vi "IMAQ_symmetrytransform_evenodd.vi"(4 "Destructive":bool, 5 "Optional Rectangle":i32[](array[numeric]), 6 "error in (no error)":errorcluster, 7 "margin":i32=15, 9 "Image Src":T1) -> (0 "error out":errorcluster, 2 "Centroid":cluster{"X Centroid":sgl, "Y Centroid":sgl} {"Y Centroid" format="%.2f"; "X Centroid" format="%.2f"}, 3 "Image Src Dup":T1)   [LabVIEW 2010]
uses:
  <vilib>/vision/Image Controls.llb/IMAQ Image.ctl
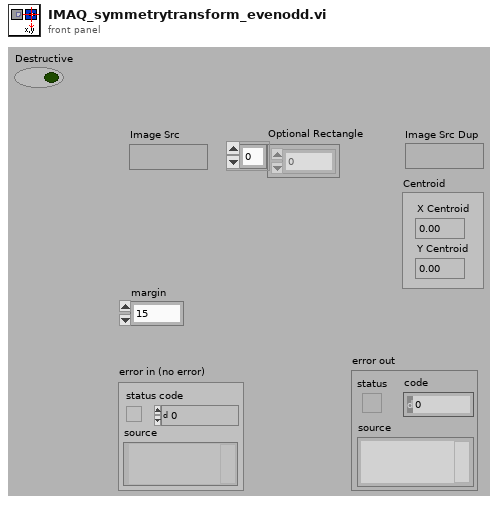
[diagram p1: front panel]
types:
  T1 = typedef "IMAQ Image.ctl" = refnum<image>
  T2 = enum32{"Map Pixel Pointer", "Unmap Pixel Pointer", "Get Pixels Infos"}
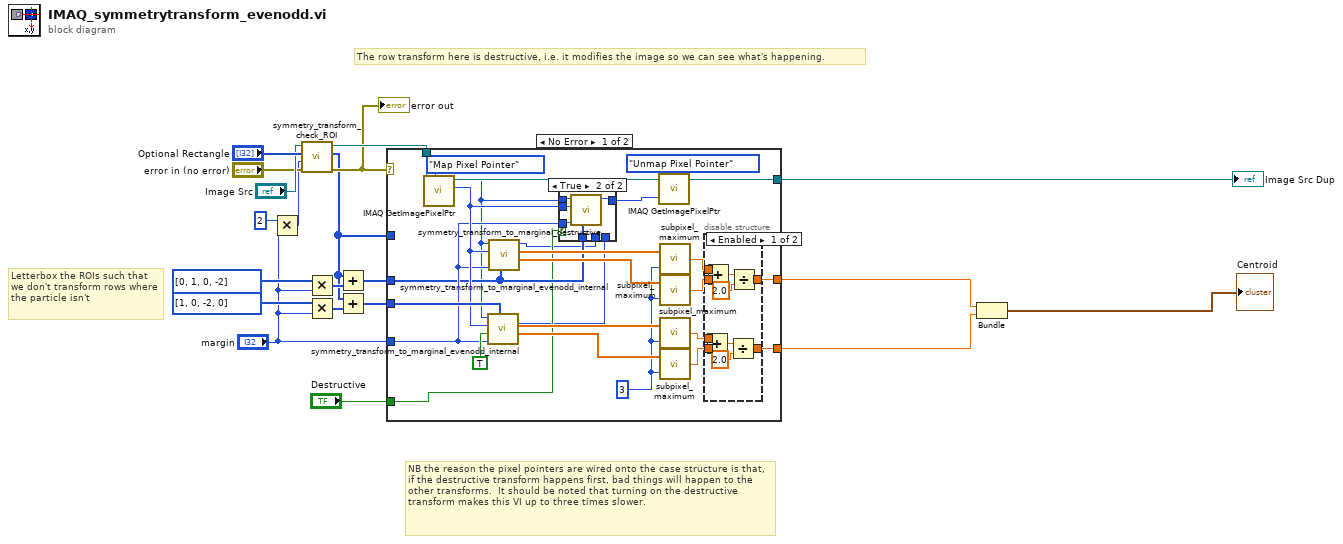
[diagram p0: block diagram]
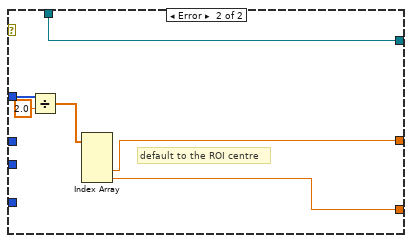
[diagram p4: hidden frame]
diagram:
  # "NB the reason the pixel pointers are wired onto the case structure is that, if the destructive transform happens first, bad things will happen to the other transforms.  It should be noted that turning on the destructive transform makes this VI up to three times slower."
  # "The row transform here is destructive, i.e. it modifies the image so we can see what's happening."
  # "Letterbox the ROIs such that we don't transform rows where the particle isn't"
  n1 = Multiply(x=2, y="margin") -> (x*y=w10:i32)
  n2 = call "symmetry_transform_check_ROI.vi"("error in (no error)"="error in (no error)", "minimum size"=w10, "Optional Rectangle"="Optional Rectangle", "Image Src"="Image Src") -> ("error out"=w8:errorcluster, "ROI Out (x,y,w,h)"=w7:i32[], "Image Src Dup"=w9:T1)  [unwired: 1 in]
  "error out" <- w8
  n3 = Multiply(x=i32[] [0, 1, 0, -2] ("Optional Rectangle"), y="margin") -> (x*y=w17:i32[])
  n4 = Multiply(x=i32[] [1, 0, -2, 0] ("Optional Rectangle"), y="margin") -> (x*y=w18:i32[])
  n5 = Add(x=w7, y=w17) -> (x+y=w16:i32[])
  n6 = Add(x=w7, y=w18) -> (x+y=w15:i32[])
  n7 = case shown="No Error" w8 {
    tunnel: [w30 w63] -> w5
    tunnel: [w29 w64] -> w4
    tunnel: w16 -> [w26 _]
    tunnel: w15 -> [w43 _]
    tunnel: w9 -> [w39 w68]
    tunnel: "margin" -> [w27 _]
    tunnel: [w39 w68] -> w3
    tunnel: w7 -> [_ w65]
    tunnel: "Destructive" -> [w24 _]
    frame No Error {
      w35 = 3 ("y")
      n8 = call "IMAQ GetImagePixelPtr"("Function"=T2."Map Pixel Pointer", "Image"=w39) -> ("LineWidth(Pixels)"=w28:i32, "Pixel Pointer out"=w22:u64)  [unwired: 4 in, 4 out]
      n9 = call "symmetry_transform_to_marginal_evenodd_internal.vi"("ROI (x,y,w,h)"=w43, "margin"=w27, "Transform Columns?"=TRUE, "LineWidth(Pixels)"=w28, "Pixel Pointer"=w22) -> ("Marginal (halfpixels)"=w36:sgl[], "Marginal"=w37:sgl[], "Pixel Pointer out"=w23:u64)  [unwired: 1 out]
      n10 = call "symmetry_transform_to_marginal_evenodd_internal.vi"("ROI (x,y,w,h)"=w26, "margin"=w27, "LineWidth(Pixels)"=w28, "Pixel Pointer"=w22) -> ("Marginal (halfpixels)"=w38:sgl[], "Marginal"=w44:sgl[], "Pixel Pointer out"=w21:u64)  [unwired: 2 in]
      n11 = case shown="True" w24 {
        tunnel: w22 -> [w45 w50]
        tunnel: w28 -> [_ w49]
        tunnel: w27 -> [_ w48]
        tunnel: w26 -> [_ w47]
        tunnel: [w45 w46] -> w25
        tunnel: w23 -> [_ _]
        tunnel: w21 -> [_ _]
        frame False {
        }
        frame True {
          n12 = call "symmetry_transform_to_marginal_destructive.vi"("ROI (x,y,w,h)"=w47, "margin"=w48, "LineWidth(Pixels)"=w49, "Pixel Pointer"=w50) -> ("Pixel Pointer out"=w46:u64)  [unwired: 3 in, 1 out]
        }
      }
      n13 = call "IMAQ GetImagePixelPtr"("Pixel Pointer in"=w25, "Function"=T2."Unmap Pixel Pointer", "Image"=w39) -> ()  [unwired: 3 in, 6 out]
      n14 = call "subpixel_maximum.vi"("Padding"=w35, "Marginal"=w44) -> ("Maximum"=w34:dbl)
      n15 = call "subpixel_maximum.vi"("Padding"=w35, "Marginal"=w38) -> ("Maximum"=w33:dbl)
      n16 = call "subpixel_maximum.vi"("Padding"=w35, "Marginal"=w37) -> ("Maximum"=w32:dbl)
      n17 = call "subpixel_maximum.vi"("Padding"=w35, "Marginal"=w36) -> ("Maximum"=w31:dbl)
      n18 = disable-structure shown="Enabled" {
        disable-tunnel: w34 -> [w60 w62]
        disable-tunnel: w33 -> [w59 _]
        disable-tunnel: w32 -> [w54 w61]
        disable-tunnel: w31 -> [w53 _]
        disable-tunnel: [w52 w62] -> w30
        disable-tunnel: [w51 w61] -> w29
        frame Enabled {
          n19 = Add(x=w54, y=w53) -> (x+y=w56:dbl)
          n20 = Add(x=w60, y=w59) -> (x+y=w57:dbl)
          n21 = Divide(x=w56, y=2.0) -> (x/y=w51:dbl)
          n22 = Divide(x=w57, y=2.0) -> (x/y=w52:dbl)
        }
        frame Disabled {
        }
      }
    }
    frame Error {
      # "default to the ROI centre"
      n23 = Divide(x=w65, y=2.0) -> (x/y=w67:dbl[])
      n24 = Index Array(array=w67) -> (element #3=w63:dbl, element #4=w64:dbl)  [unwired: 4 in, 2 out]
    }
  }
  "Image Src Dup" <- w3
  n25 = Bundle(w5, w4) -> (→"Centroid":cluster{dbl, dbl})  [unwired: 1 out]
